vi "test_ValidEnumsInConfigAndResults_ValidateMetadata_NoError.vi"(8 "error in":errorcluster) -> (0 "error out":errorcluster, 2 "result":string, 3 "pass":bool)   [LabVIEW 2020, in "MeasurementServerTests.lvlib" / "Measurement Plugin Service Tests.lvlib"]
uses:
  Measurement Plugin Service Tests.lvlib
  Fake Measurement Plugin/Fake Measurement Plugin.lvclass
  Measurement IO Enum Legal Characters.ctl
  Get Type Specializations Default.vi
  Fake Measurement Plugin/Plugin VI and Control References.ctl
  Runtime/Measurements/Measurement Plugin Measurement Server/Measurement Plugin Measurement Server.lvlib
  C:/dev/measurementlink-labview/Source/Runtime/Measurements/Measurement Plugin Measurement Server/Measurement Plugin Service/Measurement Plugin Service.lvclass
  C:/dev/measurementlink-labview/Source/Tests/Tests.Runtime/Measurement Server/Measurement Plugin Service/Fake Measurement Plugin/Fake Measurement Plugin.lvclass
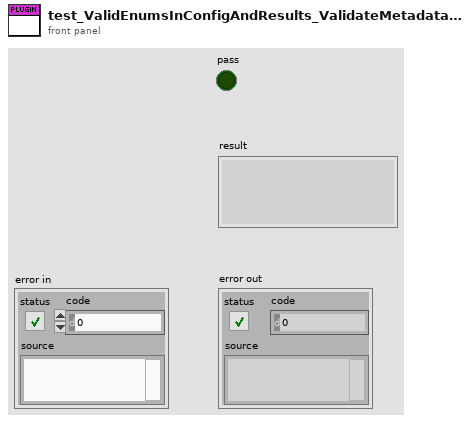
[diagram p1: front panel]
types:
  T1 = typedef "MeasurementServerTests.lvlib/Measurement Plugin Service Tests.lvlib/Fake Measurement Plugin.lvclass/Plugin VI and Control References.ctl" = cluster{"get measurement details VI ref":refnum<vi>, "get type specializations VI ref":refnum<vi>, "get UI details VI ref":refnum<vi>, "measurement logic VI ref":refnum<vi>, "measurement configuration ctl ref":refnum<vi>, "measurement results ctl path":refnum<vi>}
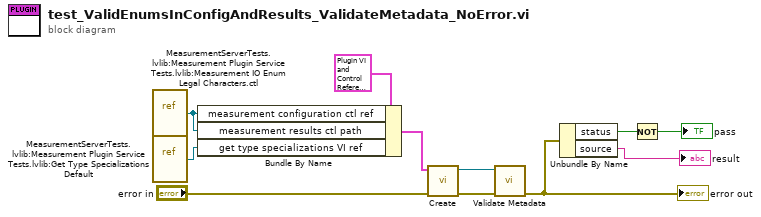
[diagram p0: block diagram]
diagram:
  n1 = vi-ref "MeasurementServerTests.lvlib:Measurement Plugin Service Tests.lvlib:Measurement IO Enum Legal Characters.ctl"() -> (w6:refnum<vi>)
  n2 = vi-ref "MeasurementServerTests.lvlib:Measurement Plugin Service Tests.lvlib:Get Type Specializations Default.vi"() -> (w7:refnum<vi>)
  n3 = Bundle By Name(cluster=T1 {"get measurement details VI ref"=refnum, "get type specializations VI ref"=refnum, "get UI details VI ref"=refnum, "measurement logic VI ref"=refnum, "measurement configuration ctl ref"=refnum, "measurement results ctl path"=refnum} ("plugin references"), "measurement configuration ctl ref"=w6, "measurement results ctl path"=w6, "get type specializations VI ref"=w7) -> (w5:T1)
  n4 = call "Create.vi"("error in"="error in", "plugin references"=w5) -> ("error out"=w3:errorcluster, "fake measurement plugin"=w4:refnum<class "Fake Measurement Plugin.lvclass">)  [unwired: 8 in]
  n5 = call "Validate Metadata.vi"("error in"=w3, "measurement plugin service in"=w4) -> ("error out"=w1:errorcluster)  [unwired: 8 in, 1 out]
  "error out" <- w1
  n6 = Unbundle By Name(w1) -> ("status"=w11:bool, "source"=→"result":string)
  n7 = Not(x=w11) -> (.not. x?=→"pass":bool)
